vi "updateIN-OUT.vi"(8 "error in (no error)":errorcluster, 9 "IN-OUT":bool, 10 "dataIN":string[][](array[string]), 11 "reference in":refnum<class "Items Controller.lvclass">) -> (0 "error out":errorcluster, 3 "reference out":refnum<class "Items Controller.lvclass">)   [LabVIEW 2016, in "Items Controller.lvclass"]
uses:
  Items Controller.lvclass
  APP/checkIN_class/checkIN.lvclass
  APP/checkOUT_class/checkOUT.lvclass
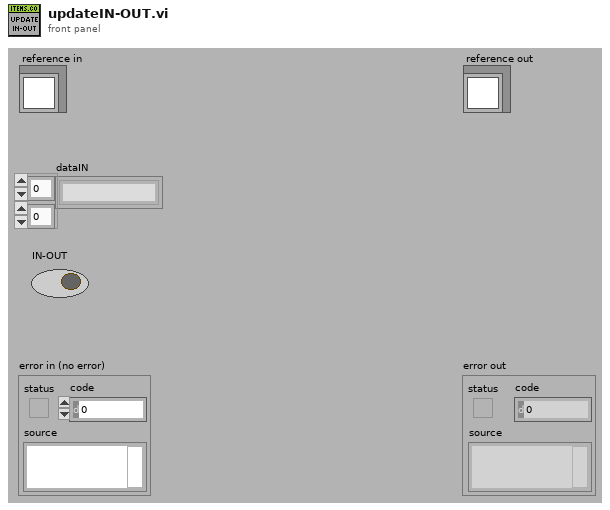
[diagram p1: front panel]
types:
  T1 = typedef "Items Controller.lvclass/ObjectAttributesRef.ctl" = refnum<data-value>
  T2 = typedef "Items Controller.lvclass/ObjectAttributes.ctl" = cluster{"MyAttribute":dbl, "data":string[][][], "file_controller_ref":refnum<class "File Controller.lvclass">, "checkIN_ref":refnum<class "checkIN.lvclass">, "checkOUT_ref":refnum<class "checkOUT.lvclass">, "item_ref":refnum<class "item.lvclass">}
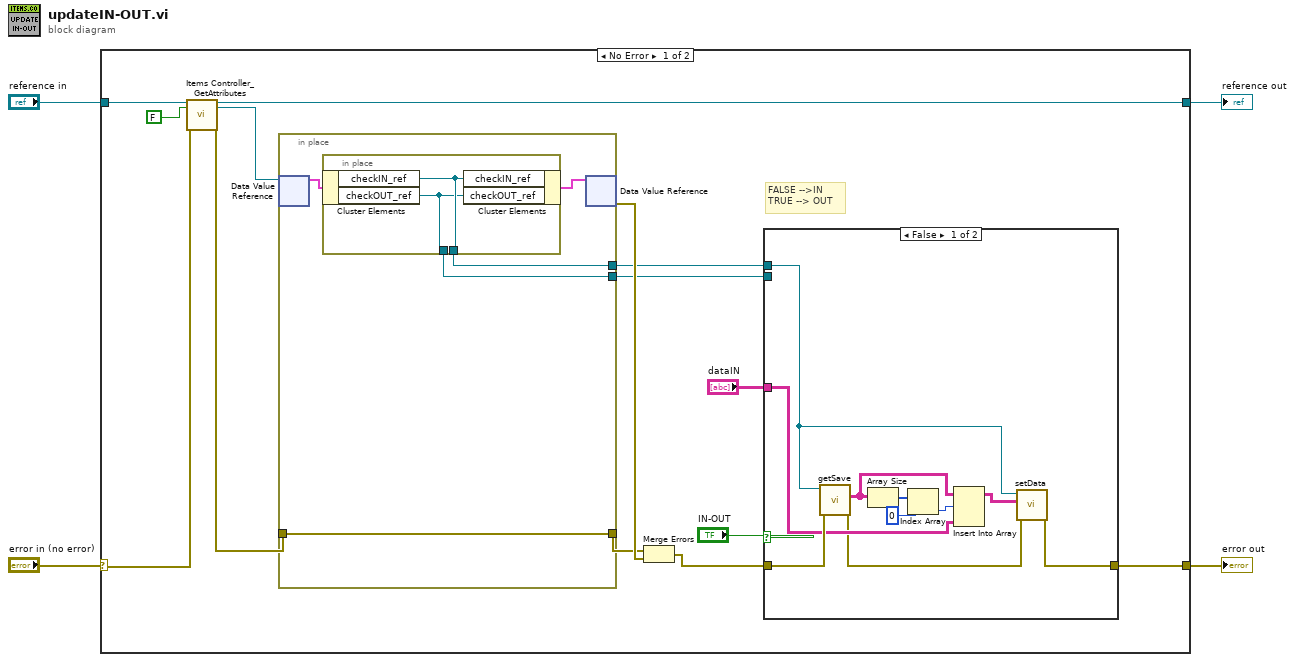
[diagram p0: block diagram]
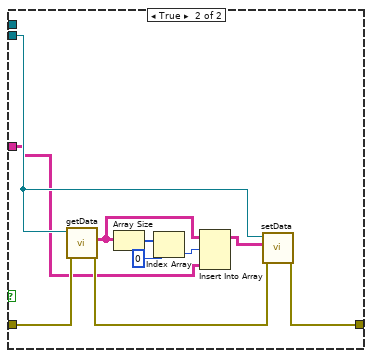
[diagram p2: hidden frame]
diagram:
  n1 = case shown="No Error" "error in (no error)" {
    selector: "error in (no error)" -> [w14 w47]
    tunnel: [w5 w47] -> w3
    tunnel: [w12 w46] -> w1
    tunnel: "reference in" -> [w16 w46]
    frame No Error {
      # "FALSE -->IN\nTRUE --> OUT"
      n2 = call "Items Controller_GetAttributes.vi"("reference in"=w16, "return data? (T)"=FALSE, "error in (no error)"=w14) -> ("reference out"=w12:refnum<class "Items Controller.lvclass">, "attributes ref"=w11:T1, "error out"=w13:errorcluster)  [unwired: 13 in, 1 out]
      n3 = in-place {
        in-place-border: w13 -> [w41]
        in-place-border: [w41] -> w17
        in-place-border: [w40] -> w7
        in-place-border: [w39] -> w6
        n4 = in-place-dvr #1(w11) -> (w42:T2)  [unwired: 1 out]
        n5 = in-place {
          in-place-border: [w45] -> w40
          in-place-border: [w44] -> w39
          n6 = in-place-cluster #2(w42) -> ("checkIN_ref"=w45:refnum<class "checkIN.lvclass">, "checkOUT_ref"=w44:refnum<class "checkOUT.lvclass">)
          n7 = in-place-cluster #2("checkIN_ref"=w45, "checkOUT_ref"=w44) -> (w43:T2)
        }
        n8 = in-place-dvr #1(w43) -> (w18:errorcluster)  [unwired: 1 out]
      }
      n9 = Merge Errors(w17, w18) -> (w10:errorcluster)
      n10 = case shown="False" "IN-OUT" {
        tunnel: w10 -> [w28 w33]
        tunnel: [w19 w31] -> w5
        tunnel: "dataIN" -> [w26 w29]
        tunnel: w7 -> [w21 _]
        tunnel: w6 -> [_ w30]
        frame False {
          n11 = call "getSave.vi"("error in (no error)"=w28, "reference in"=w21) -> ("error out"=w20:errorcluster, "data"=w27:string[][])  [unwired: 7 in, 1 out]
          n12 = Array Size(array=w27) -> (size(s)=w25:i32[])
          n13 = Index Array(array=w25, index=0) -> (element=w24:i32)
          n14 = Insert Into Array(array=w27, index (row)=w24, new element=w26) -> (w22:string[][])  [unwired: 1 in]
          n15 = call "setData.vi"("error in (no error)"=w20, "data"=w22, "reference in"=w21) -> ("error out"=w19:errorcluster)  [unwired: 7 in, 1 out]
        }
        frame True {
          n16 = call "getData.vi"("error in (no error)"=w33, "reference in"=w30) -> ("error out"=w32:errorcluster, "data"=w38:string[][])  [unwired: 7 in, 1 out]
          n17 = Array Size(array=w38) -> (size(s)=w37:i32[])
          n18 = Index Array(array=w37, index=0) -> (element=w36:i32)
          n19 = Insert Into Array(array=w38, index (row)=w36, new element=w29) -> (w34:string[][])  [unwired: 1 in]
          n20 = call "setData.vi"("error in (no error)"=w32, "data"=w34, "reference in"=w30) -> ("error out"=w31:errorcluster)  [unwired: 7 in, 1 out]
        }
      }
    }
    frame Error {
    }
  }
  "error out" <- w3
  "reference out" <- w1
